vi "BotSpeak_DIORead.vi"(2 "Bot Settings":T1, 3 "DIO Line":u32) -> (1 "State":bool, 4 "Bot Settings out":T1)   [LabVIEW 2012]
doc: "Reads the value of the DIO pin specified by \"DIO Line\" and outputs the boolean \"State\" of the line."
uses:
  <userlib>/botspeak/VIs/Direct/BotSpeak_Control.ctl
panel:
  out "response":string
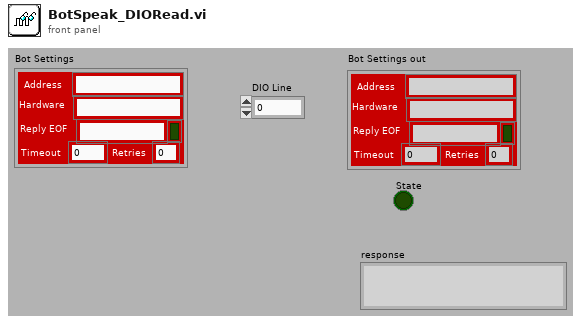
[diagram p1: front panel]
types:
  T1 = typedef "BotSpeak_Control.ctl" = cluster{"Address":string, "Reply EOF":string, "Hardware":string, "Retries":i8, "Timeout":i32, "Open?":bool}
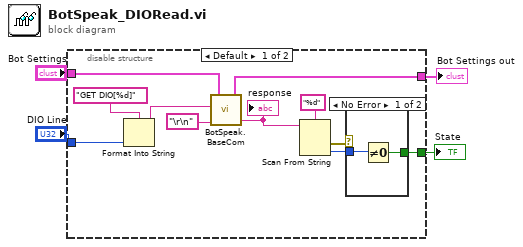
[diagram p0: block diagram]
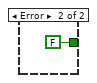
[diagram p2: hidden frame]
diagram:
  n1 = disable-structure shown="Default" {
    disable-tunnel: "Bot Settings" -> [w14 _]
    disable-tunnel: [w11 _] -> w3
    disable-tunnel: "DIO Line" -> [w10 _]
    disable-tunnel: [w8 _] -> w1
    frame condition #0 (active) {
      n2 = Format Into String(format string="GET DIO[%d]" ("command"), w10) -> (resulting string=w13:string)  [unwired: 2 in, 1 out]
      n3 = call <userlib>:"BotSpeak.BaseCom.vi"("Termination"="\r\n", "command"=w13, "Bot Settings in"=w14) -> ("response"=w6:string, "Bot Settings out"=w11:T1)  [unwired: 2 in]
      "response" <- w6
      n4 = Scan From String(format string="%d", input string=w6) -> (error out=w7:errorcluster, output 1=w9:i32)  [unwired: 3 in, 2 out]
      n5 = case shown="No Error" w7 {
        tunnel: w9 -> [w17 _]
        tunnel: [w16 FALSE] -> w8
        frame No Error {
          n6 = Not Equal To 0?(x=w17) -> (x != 0?=w16:bool)
        }
        frame Error {
        }
      }
    }
    frame condition #1 {
      # "Add in response and make \n255 = True, 0 = False for the ev3"
    }
  }
  "State" <- w1
  "Bot Settings out" <- w3
